vi "update safe outputs.vi"(9 "Message handler data":T1, 11 "Data":variant) -> (0 "error":errorcluster)   [LabVIEW 2018]
uses:
  Type Defs/Message loop data.ctl
  Type Defs/FPGA reference.ctl
  Type Defs/RT Status.ctl
  <vilib>/Utility/error.llb/Error Cluster From Error Code.vi
  <vilib>/rvi/errors/niLvFpgaAdjustHostInterfaceError.vi
  <vilib>/rvi/interface/nirviReadWriteControl/nirviReadWriteControl.xnode
  FPGA Bitfiles/CompressorRigV2_CompressorFPGA_FPGAMainV3_7sPRekuravM.lvbitx
  NiFpgaLv.dll
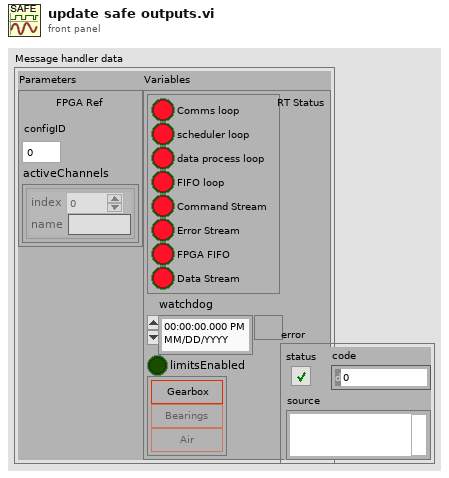
[diagram p1: front panel]
types:
  T1 = typedef "Message loop data.ctl" = cluster{"Parameters":cluster{"FPGA Ref":T2, "configID":u32, "activeChannels":cluster{"index":u16, "name":string}[]}, "Variables":cluster{"RT Status":T3, "watchdog":timestamp, "limitsEnabled":bool, "Interlocks":cluster{"gearboxOil":bool, "bearingOil":bool, "gearboxAir":bool}}}
  T2 = typedef "FPGA reference.ctl" = refnum<k20>
  T3 = typedef "RT Status.ctl" = cluster{"Comms loop":bool, "scheduler loop":bool, "data process loop":bool, "FIFO loop":bool, "Command Stream":bool, "Error Stream":bool, "FPGA FIFO":bool, "Data Stream":bool}
  T4 = cluster{"Safe Digital":bool[], "Safe Voltage":fxp<+/-,20,5>[]}
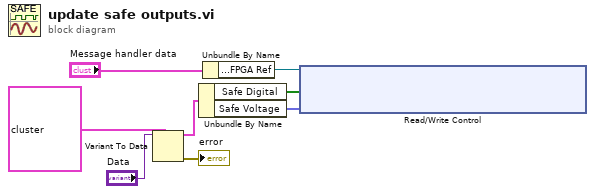
[diagram p0: block diagram]
diagram:
  n1 = Variant To Data(type=T4 {"Safe Digital"=[FALSE, FALSE, FALSE, FALSE, FALSE, FALSE, FALSE, FALSE], "Safe Voltage"=[0.0, 0.0, 0.0, 0.0]}, Variant="Data") -> (data=w4:T4, error out=→"error":errorcluster)  [unwired: 1 in]
  n2 = Unbundle By Name(w4) -> ("Safe Digital"=w2:bool[], "Safe Voltage"=w1:fxp<+/-,20,5>[])
  n3 = Unbundle By Name("Message handler data") -> ("Parameters.FPGA Ref"=w7:T2)
  n4 = xnode "Read/Write Control"("FPGA VI Reference In"=w7, "Safe Digital"=w2, "Safe Voltage"=w1) -> ()  [unwired: 1 in, 2 out]
